vi "Read.vi"(8 "error in (no error)":errorcluster, 11 "DAQmx in":refnum<class "DAQmx.lvclass">) -> (0 "error out":errorcluster, 2 "Output":variant, 3 "DAQmx out":refnum<class "DAQmx.lvclass">)   [LabVIEW 2017, in "DAQmx.lvclass"]
uses:
  DAQmx.lvclass
  Generic/Generic Hardware.lvclass
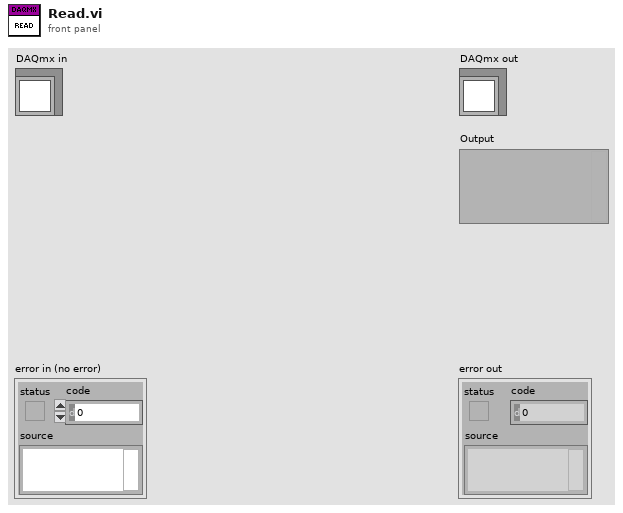
[diagram p1: front panel]
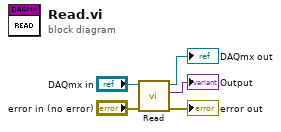
[diagram p0: block diagram]
diagram:
  n1 = call-parent "Read.vi"("error in (no error)"="error in (no error)", "Generic Hardware in"="DAQmx in") -> ("error out"=→"error out":errorcluster, "Output"=→"Output":variant, "Generic Hardware out"=→"DAQmx out":refnum<class "DAQmx.lvclass">)  [unwired: 7 in]
